vi "Read Measurement (Channel Power).vi"(0 "VISA resource name":refnum<visa-resource-name>, 11 "error in (no error)":errorcluster) -> (4 "VISA resource name out":refnum<visa-resource-name>, 6 "Channel Power Measurement":T1, 15 "error out":errorcluster)   [LabVIEW 2020, in "Anritsu Signal Analyzer Series.lvlib"]
doc: "Reads Channel Power measurement data"
uses:
  Anritsu Signal Analyzer Series.lvlib
panel:
  # "Hz"
  # "dBm"
  # "Hz"
  # "dBm/"
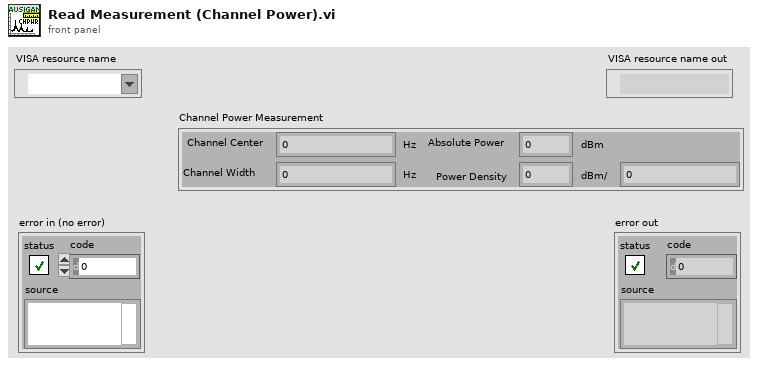
[diagram p1: front panel]
types:
  T1 = cluster{"Channel Center":dbl, "Channel Width":dbl, "Absolute Power":dbl, "Power Density":dbl, "Channel Width 2":dbl}
  T2 = cluster{"[0]":dbl, "[1]":dbl, "[2]":dbl, "[3]":dbl, "[4]":dbl}
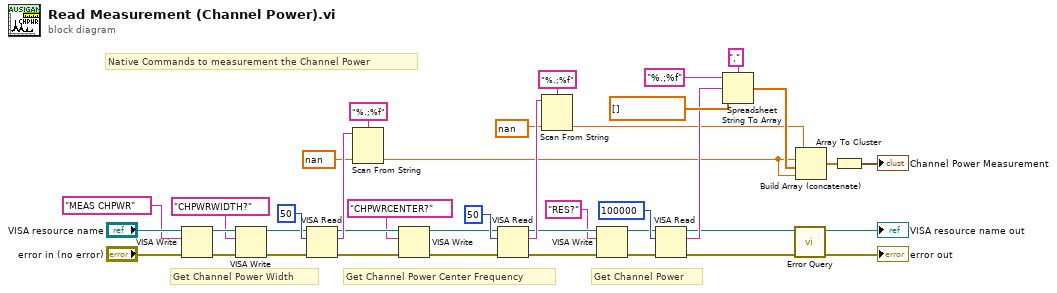
[diagram p0: block diagram]
diagram:
  # "Get Channel Power Width"
  # "Get Channel Power"
  # "Get Channel Power Center Frequency"
  # "Native Commands to measurement the Channel Power"
  n1 = VISA Write(VISA resource name="VISA resource name", write buffer="MEAS CHPWR" ("_CommandSet"), error in (no error)="error in (no error)") -> (VISA resource name out=w29:refnum<visa-resource-name>, error out=w28:errorcluster)  [unwired: 1 out]
  n2 = VISA Write(VISA resource name=w29, write buffer="CHPWRWIDTH?" ("_CommandGet"), error in (no error)=w28) -> (VISA resource name out=w30:refnum<visa-resource-name>, error out=w31:errorcluster)  [unwired: 1 out]
  n3 = VISA Read(VISA resource name=w30, byte count=u32 50 ("byte count (0)"), error in (no error)=w31) -> (VISA resource name out=w21:refnum<visa-resource-name>, read buffer=w33:string, error out=w20:errorcluster)  [unwired: 1 out]
  n4 = Scan From String(format string="%.;%f" ("Format String"), input string=w33, default 1=nan) -> (output 1=w1:dbl)  [unwired: 2 in, 3 out]
  n5 = VISA Write(VISA resource name=w21, write buffer="CHPWRCENTER?" ("_CommandGet"), error in (no error)=w20) -> (VISA resource name out=w22:refnum<visa-resource-name>, error out=w23:errorcluster)  [unwired: 1 out]
  n6 = VISA Read(VISA resource name=w22, byte count=u32 50 ("byte count (0)"), error in (no error)=w23) -> (VISA resource name out=w11:refnum<visa-resource-name>, read buffer=w25:string, error out=w10:errorcluster)  [unwired: 1 out]
  n7 = Scan From String(format string="%.;%f" ("Format String"), input string=w25, default 1=nan) -> (output 1=w2:dbl)  [unwired: 2 in, 3 out]
  n8 = VISA Write(VISA resource name=w11, write buffer="RES?" ("_Command"), error in (no error)=w10) -> (VISA resource name out=w12:refnum<visa-resource-name>, error out=w13:errorcluster)  [unwired: 1 out]
  n9 = VISA Read(VISA resource name=w12, byte count=u32 100000 ("byte count (0)"), error in (no error)=w13) -> (VISA resource name out=w9:refnum<visa-resource-name>, read buffer=w17:string, error out=w8:errorcluster)  [unwired: 1 out]
  n10 = Spreadsheet String To Array(delimiter (Tab)=",", format string="%.;%f", spreadsheet string=w17, array type (2D Dbl)=dbl[] [] ("Values")) -> (array=w7:dbl[])
  n11 = call "Error Query.vi"("error in (no error)"=w8, "VISA resource name"=w9) -> ("error out"=→"error out":errorcluster, "VISA resource name out"=→"VISA resource name out":refnum<visa-resource-name>)  [unwired: 6 in, 2 out]
  n12 = Build Array (concatenate)(w2, w1, w7, w1) -> (w35:dbl[])
  n13 = Array To Cluster(array=w35) -> (cluster=→"Channel Power Measurement":T2)
